vi "Move and Merge Element.vi"(7 "Direction":T2, 11 "Board Array":u8[][](array[numeric])) -> (1 "Game Status":T1, 2 "Score":i32, 3 "Board Array":u8[][](array[numeric]))   [LabVIEW 2020, in "Game.lvlib"]
uses:
  Game.lvlib
  Direction.ctl
  Game Status.ctl
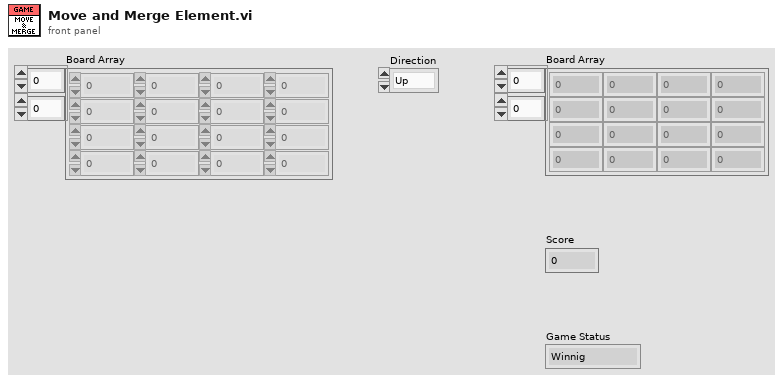
[diagram p1: front panel]
types:
  T1 = typedef "Game Status.ctl" = enum16{"Winnig", "Game Over", "Continute"}
  T2 = typedef "Direction.ctl" = enum16{"Up", "Down", "Left", "Right"}
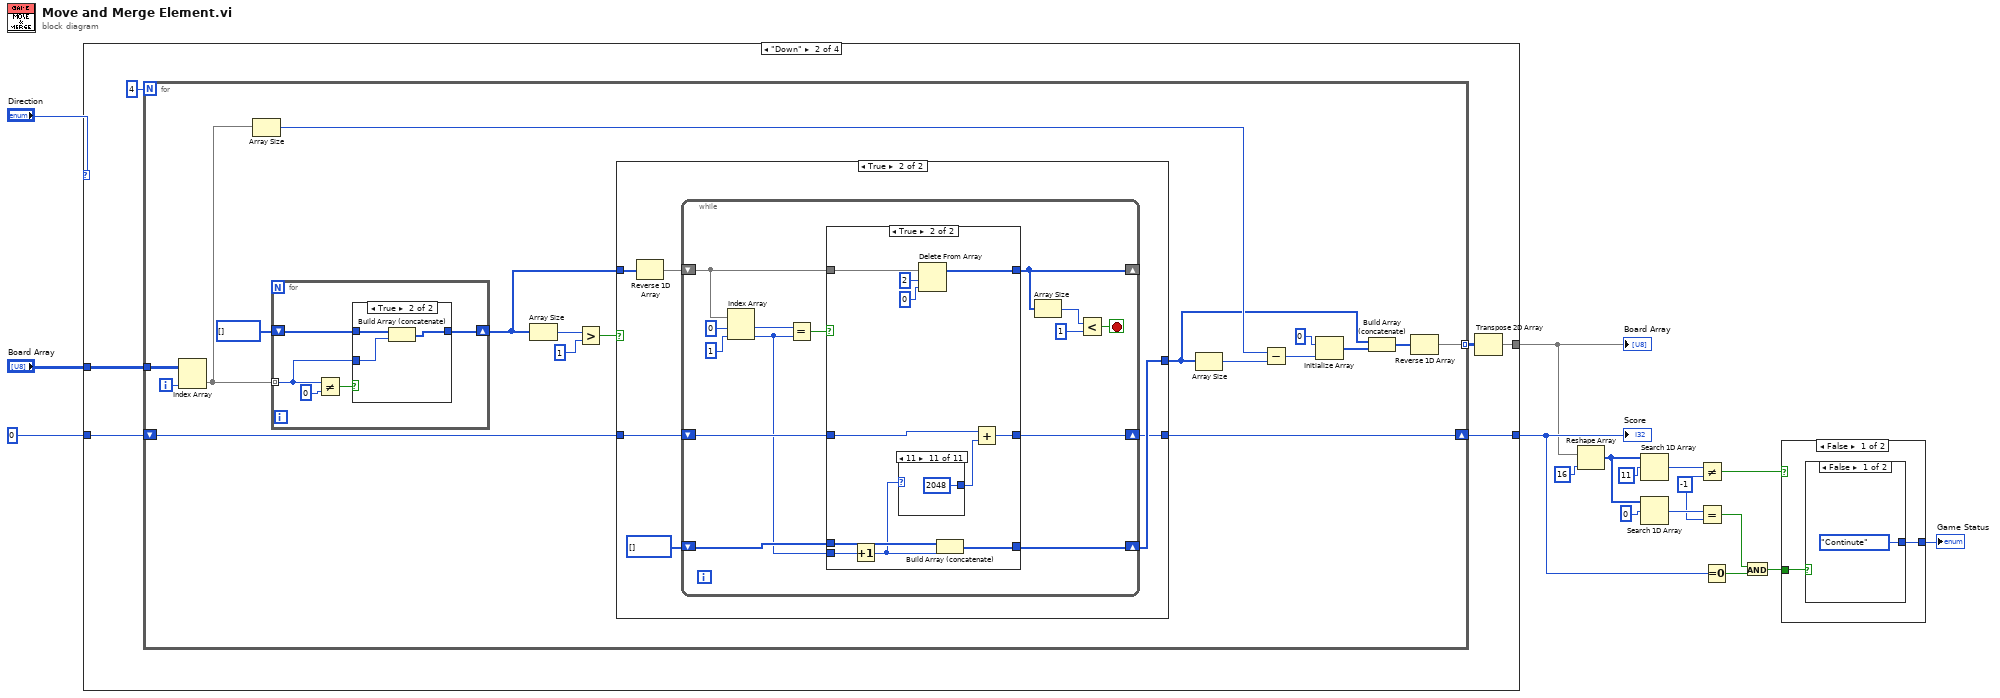
[diagram p0: block diagram]
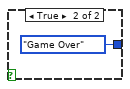
[diagram p2: hidden frame]
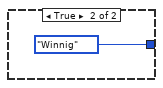
[diagram p3: hidden frame]
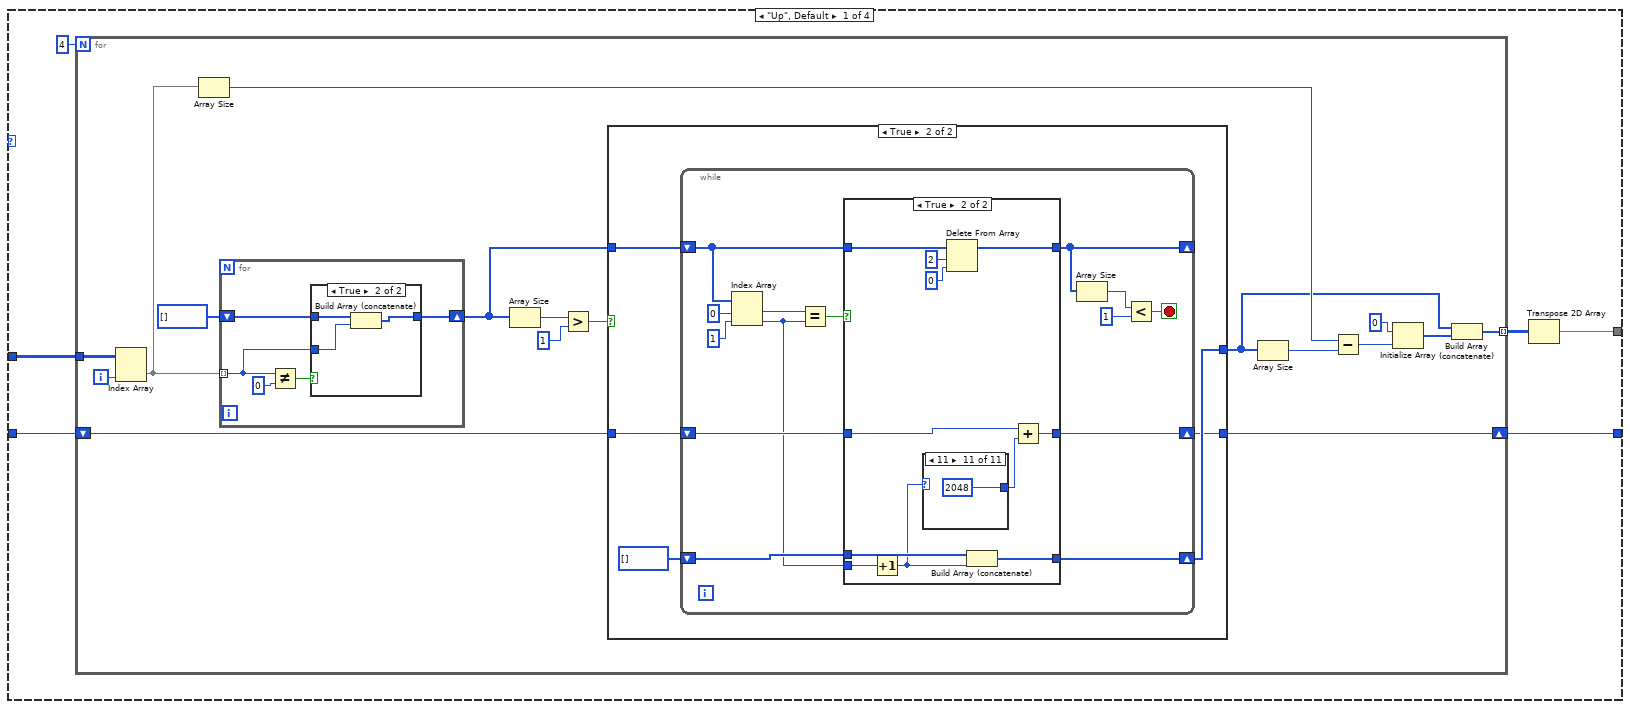
[diagram p4: hidden frame]
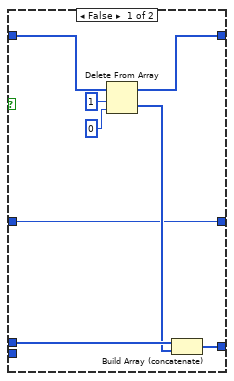
[diagram p6: hidden frame]
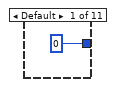
[diagram p7: hidden frame]
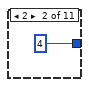
[diagram p8: hidden frame]
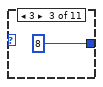
[diagram p9: hidden frame]
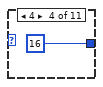
[diagram p10: hidden frame]
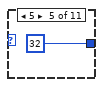
[diagram p11: hidden frame]
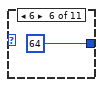
[diagram p12: hidden frame]
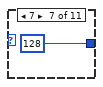
[diagram p13: hidden frame]
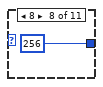
[diagram p14: hidden frame]
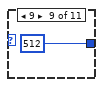
[diagram p15: hidden frame]
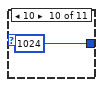
[diagram p16: hidden frame]
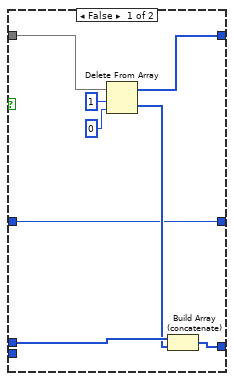
[diagram p19: hidden frame]
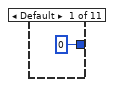
[diagram p20: hidden frame]
diagram:
  w1 = -1 ("y")
  n1 = case shown="\"Down\"" "Direction" {
    tunnel: "Board Array" -> [w23 w106 w190 w272]
    tunnel: [w18 w101 w188 w270] -> w2
    tunnel: [w20 w103 w187 w269] -> w13
    tunnel: 0 -> [w19 w102 w186 w268]
    frame "Up", Default {
      n2 = for {
        N: 4 -> [_]
        tunnel: w23 -> [w40]
        tunnel: [w25] -> w21 mode=indexing
        shift-right: [w28] -> w20
        shift-left: w19 -> [w27]
        i -> [w26]
        n3 = Index Array(array=w40, index (col)=w26) -> (element=w38:u8[])  [unwired: 1 in]
        n4 = Array Size(array=w38) -> (size(s)=w37:i32)
        n5 = for {
          tunnel: w38 -> [w94] mode=indexing
          shift-right: [w93] -> w32
          shift-left: u8[] [] -> [w92]
          n6 = Not Equal?(x=w94, y=u8 0) -> (x != y?=w95:bool)
          n7 = case shown="True" w95 {
            tunnel: w94 -> [_ w98]
            tunnel: [w97 w100] -> w93
            tunnel: w92 -> [w97 w99]
            frame False {
            }
            frame True {
              n8 = Build Array (concatenate)(w99, w98) -> (w100:u8[])
            }
          }
        }
        n9 = Array Size(array=w32) -> (size(s)=w31:i32)
        n10 = Greater?(x=w31, y=1) -> (0:w33:bool)
        n11 = case shown="True" w33 {
          tunnel: w32 -> [w42 w45]
          tunnel: [w42 w46] -> w30
          tunnel: [w41 w44] -> w28
          tunnel: w27 -> [w41 w43]
          frame False {
          }
          frame True {
            n12 = while {
              shift-right: [w48] -> _
              shift-left: w45 -> [w60]
              shift-right: [w56] -> w46
              shift-left: u8[] [] -> [w55]
              shift-right: [w51] -> w44
              shift-left: w43 -> [w50]
              stop <- w54 stop-if-true
              n13 = Index Array(array=w60, index #1=0 ("index"), index #2=1 ("index")) -> (element #1=w59:u8, element #2=w49:u8)
              n14 = Equal?(x=w59, y=w49) -> (x = y?=w61:bool)
              n15 = case shown="True" w61 {
                tunnel: w60 -> [w69 w79]
                tunnel: [w66 w76] -> w48
                tunnel: w49 -> [_ w80]
                tunnel: [w65 w75] -> w56
                tunnel: w55 -> [w64 w74]
                tunnel: [w62 w72] -> w51
                tunnel: w50 -> [w62 w73]
                frame False {
                  n16 = Delete From Array(array=w69, length=1, index=0) -> (deleted portion=w63:u8[], array with subset deleted=w66:u8[])
                  n17 = Build Array (concatenate)(w64, w63) -> (w65:u8[])
                }
                frame True {
                  n18 = Increment(x=w80) -> (x+1=w70:u8)
                  n19 = case shown="11" w70 {
                    tunnel: [0 4 8 16 32 64 128 256 512 1024 2048] -> w71
                    frame Default {
                    }
                    frame 2 {
                    }
                    frame 3 {
                    }
                    frame 4 {
                    }
                    frame 5 {
                    }
                    frame 6 {
                    }
                    frame 7 {
                    }
                    frame 8 {
                    }
                    frame 9 {
                    }
                    frame 10 {
                    }
                    frame 11 {
                    }
                  }
                  n20 = Delete From Array(array=w79, length=2, index=0) -> (array with subset deleted=w76:u8[])  [unwired: 1 out]
                  n21 = Build Array (concatenate)(w74, w70) -> (w75:u8[])
                  n22 = Add(x=w73, y=w71) -> (x+y=w72:i32)
                }
              }
              n23 = Array Size(array=w48) -> (size(s)=w52:i32)
              n24 = Less?(x=w52, y=1) -> (x < y?=w54:bool)
            }
          }
        }
        n25 = Array Size(array=w30) -> (size(s)=w24:i32)
        n26 = Subtract(x=w37, y=w24) -> (x-y=w29:i32)
        n27 = Initialize Array(u8 0, w29) -> (w35:u8[])
        n28 = Build Array (concatenate)(w30, w35) -> (w25:u8[])
      }
      n29 = Transpose 2D Array(2D array=w21) -> (transposed array=w18:u8[][])
    }
    frame "Down" {
      n30 = for {
        N: 4 -> [_]
        tunnel: w106 -> [w124]
        tunnel: [w111] -> w104 mode=indexing
        shift-right: [w110] -> w103
        shift-left: w102 -> [w109]
        i -> [w108]
        n31 = Index Array(array=w124, index (col)=w108) -> (element=w122:u8[])  [unwired: 1 in]
        n32 = Array Size(array=w122) -> (size(s)=w121:i32)
        n33 = for {
          tunnel: w122 -> [w179] mode=indexing
          shift-right: [w178] -> w116
          shift-left: u8[] [] -> [w177]
          n34 = Not Equal?(x=w179, y=u8 0) -> (x != y?=w180:bool)
          n35 = case shown="True" w180 {
            tunnel: w179 -> [_ w183]
            tunnel: [w182 w185] -> w178
            tunnel: w177 -> [w182 w184]
            frame False {
            }
            frame True {
              n36 = Build Array (concatenate)(w184, w183) -> (w185:u8[])
            }
          }
        }
        n37 = Array Size(array=w116) -> (size(s)=w115:i32)
        n38 = Greater?(x=w115, y=1) -> (0:w117:bool)
        n39 = case shown="True" w117 {
          tunnel: w116 -> [w126 w131]
          tunnel: [w126 w130] -> w114
          tunnel: [w125 w128] -> w110
          tunnel: w109 -> [w125 w127]
          frame False {
          }
          frame True {
            n40 = Reverse 1D Array(array=w131) -> (reversed array=w129:u8[])
            n41 = while {
              shift-right: [w133] -> _
              shift-left: w129 -> [w145]
              shift-right: [w141] -> w130
              shift-left: u8[] [] -> [w140]
              shift-right: [w136] -> w128
              shift-left: w127 -> [w135]
              stop <- w139 stop-if-true
              n42 = Index Array(array=w145, index #1=0 ("index"), index #2=1 ("index")) -> (element #1=w144:u8, element #2=w134:u8)
              n43 = Equal?(x=w144, y=w134) -> (x = y?=w146:bool)
              n44 = case shown="True" w146 {
                tunnel: w145 -> [w154 w164]
                tunnel: [w151 w161] -> w133
                tunnel: w134 -> [_ w165]
                tunnel: [w150 w160] -> w141
                tunnel: w140 -> [w149 w159]
                tunnel: [w147 w157] -> w136
                tunnel: w135 -> [w147 w158]
                frame False {
                  n45 = Delete From Array(array=w154, length=1, index=0) -> (deleted portion=w148:u8[], array with subset deleted=w151:u8[])
                  n46 = Build Array (concatenate)(w149, w148) -> (w150:u8[])
                }
                frame True {
                  n47 = Increment(x=w165) -> (x+1=w155:u8)
                  n48 = case shown="11" w155 {
                    tunnel: [0 4 8 16 32 64 128 256 512 1024 2048] -> w156
                    frame Default {
                    }
                    frame 2 {
                    }
                    frame 3 {
                    }
                    frame 4 {
                    }
                    frame 5 {
                    }
                    frame 6 {
                    }
                    frame 7 {
                    }
                    frame 8 {
                    }
                    frame 9 {
                    }
                    frame 10 {
                    }
                    frame 11 {
                    }
                  }
                  n49 = Delete From Array(array=w164, length=2, index=0) -> (array with subset deleted=w161:u8[])  [unwired: 1 out]
                  n50 = Build Array (concatenate)(w159, w155) -> (w160:u8[])
                  n51 = Add(x=w158, y=w156) -> (x+y=w157:i32)
                }
              }
              n52 = Array Size(array=w133) -> (size(s)=w137:i32)
              n53 = Less?(x=w137, y=1) -> (x < y?=w139:bool)
            }
          }
        }
        n54 = Array Size(array=w114) -> (size(s)=w107:i32)
        n55 = Subtract(x=w121, y=w107) -> (x-y=w113:i32)
        n56 = Initialize Array(u8 0, w113) -> (w119:u8[])
        n57 = Build Array (concatenate)(w114, w119) -> (w112:u8[])
        n58 = Reverse 1D Array(array=w112) -> (reversed array=w111:u8[])
      }
      n59 = Transpose 2D Array(2D array=w104) -> (transposed array=w101:u8[][])
    }
    frame "Left" {
      n60 = for {
        N: 4 -> [_]
        tunnel: w190 -> [w207]
        tunnel: [w194] -> w188 mode=indexing
        shift-right: [w193] -> w187
        shift-left: w186 -> [w192]
        i -> [w195]
        n61 = Index Array(array=w207, index (row)=w195) -> (element=w205:u8[])  [unwired: 1 in]
        n62 = Array Size(array=w205) -> (size(s)=w204:i32)
        n63 = for {
          tunnel: w205 -> [w261] mode=indexing
          shift-right: [w260] -> w199
          shift-left: u8[] [] -> [w259]
          n64 = Not Equal?(x=w261, y=u8 0) -> (x != y?=w262:bool)
          n65 = case shown="True" w262 {
            tunnel: w261 -> [_ w265]
            tunnel: [w264 w267] -> w260
            tunnel: w259 -> [w264 w266]
            frame False {
            }
            frame True {
              n66 = Build Array (concatenate)(w266, w265) -> (w267:u8[])
            }
          }
        }
        n67 = Array Size(array=w199) -> (size(s)=w198:i32)
        n68 = Greater?(x=w198, y=1) -> (0:w200:bool)
        n69 = case shown="True" w200 {
          tunnel: w199 -> [w209 w212]
          tunnel: [w209 w213] -> w197
          tunnel: [w208 w211] -> w193
          tunnel: w192 -> [w208 w210]
          frame False {
          }
          frame True {
            n70 = while {
              shift-right: [w215] -> _
              shift-left: w212 -> [w227]
              shift-right: [w223] -> w213
              shift-left: u8[] [] -> [w222]
              shift-right: [w218] -> w211
              shift-left: w210 -> [w217]
              stop <- w221 stop-if-true
              n71 = Index Array(array=w227, index #1=0 ("index"), index #2=1 ("index")) -> (element #1=w226:u8, element #2=w216:u8)
              n72 = Equal?(x=w226, y=w216) -> (x = y?=w228:bool)
              n73 = case shown="True" w228 {
                tunnel: w227 -> [w236 w246]
                tunnel: [w233 w243] -> w215
                tunnel: w216 -> [_ w247]
                tunnel: [w232 w242] -> w223
                tunnel: w222 -> [w231 w241]
                tunnel: [w229 w239] -> w218
                tunnel: w217 -> [w229 w240]
                frame False {
                  n74 = Delete From Array(array=w236, length=1, index=0) -> (deleted portion=w230:u8[], array with subset deleted=w233:u8[])
                  n75 = Build Array (concatenate)(w231, w230) -> (w232:u8[])
                }
                frame True {
                  n76 = Increment(x=w247) -> (x+1=w237:u8)
                  n77 = case shown="11" w237 {
                    tunnel: [0 4 8 16 32 64 128 256 512 1024 2048] -> w238
                    frame Default {
                    }
                    frame 2 {
                    }
                    frame 3 {
                    }
                    frame 4 {
                    }
                    frame 5 {
                    }
                    frame 6 {
                    }
                    frame 7 {
                    }
                    frame 8 {
                    }
                    frame 9 {
                    }
                    frame 10 {
                    }
                    frame 11 {
                    }
                  }
                  n78 = Delete From Array(array=w246, length=2, index=0) -> (array with subset deleted=w243:u8[])  [unwired: 1 out]
                  n79 = Build Array (concatenate)(w241, w237) -> (w242:u8[])
                  n80 = Add(x=w240, y=w238) -> (x+y=w239:i32)
                }
              }
              n81 = Array Size(array=w215) -> (size(s)=w219:i32)
              n82 = Less?(x=w219, y=1) -> (x < y?=w221:bool)
            }
          }
        }
        n83 = Array Size(array=w197) -> (size(s)=w191:i32)
        n84 = Subtract(x=w204, y=w191) -> (x-y=w196:i32)
        n85 = Initialize Array(u8 0, w196) -> (w202:u8[])
        n86 = Build Array (concatenate)(w197, w202) -> (w194:u8[])
      }
    }
    frame "Right" {
      n87 = for {
        N: 4 -> [_]
        tunnel: w272 -> [w290]
        tunnel: [w276] -> w270 mode=indexing
        shift-right: [w275] -> w269
        shift-left: w268 -> [w274]
        i -> [w277]
        n88 = Index Array(array=w290, index (row)=w277) -> (element=w288:u8[])  [unwired: 1 in]
        n89 = Array Size(array=w288) -> (size(s)=w287:i32)
        n90 = for {
          tunnel: w288 -> [w345] mode=indexing
          shift-right: [w344] -> w282
          shift-left: u8[] [] -> [w343]
          n91 = Not Equal?(x=w345, y=u8 0) -> (x != y?=w346:bool)
          n92 = case shown="True" w346 {
            tunnel: w345 -> [_ w349]
            tunnel: [w348 w351] -> w344
            tunnel: w343 -> [w348 w350]
            frame False {
            }
            frame True {
              n93 = Build Array (concatenate)(w350, w349) -> (w351:u8[])
            }
          }
        }
        n94 = Array Size(array=w282) -> (size(s)=w281:i32)
        n95 = Greater?(x=w281, y=1) -> (0:w283:bool)
        n96 = case shown="True" w283 {
          tunnel: w282 -> [w292 w297]
          tunnel: [w292 w296] -> w280
          tunnel: [w291 w294] -> w275
          tunnel: w274 -> [w291 w293]
          frame False {
          }
          frame True {
            n97 = Reverse 1D Array(array=w297) -> (reversed array=w295:u8[])
            n98 = while {
              shift-right: [w299] -> _
              shift-left: w295 -> [w311]
              shift-right: [w307] -> w296
              shift-left: u8[] [] -> [w306]
              shift-right: [w302] -> w294
              shift-left: w293 -> [w301]
              stop <- w305 stop-if-true
              n99 = Index Array(array=w311, index #1=0 ("index"), index #2=1 ("index")) -> (element #1=w310:u8, element #2=w300:u8)
              n100 = Equal?(x=w310, y=w300) -> (x = y?=w312:bool)
              n101 = case shown="True" w312 {
                tunnel: w311 -> [w320 w330]
                tunnel: [w317 w327] -> w299
                tunnel: w300 -> [_ w331]
                tunnel: [w316 w326] -> w307
                tunnel: w306 -> [w315 w325]
                tunnel: [w313 w323] -> w302
                tunnel: w301 -> [w313 w324]
                frame False {
                  n102 = Delete From Array(array=w320, length=1, index=0) -> (deleted portion=w314:u8[], array with subset deleted=w317:u8[])
                  n103 = Build Array (concatenate)(w315, w314) -> (w316:u8[])
                }
                frame True {
                  n104 = Increment(x=w331) -> (x+1=w321:u8)
                  n105 = case shown="11" w321 {
                    tunnel: [0 4 8 16 32 64 128 256 512 1024 2048] -> w322
                    frame Default {
                    }
                    frame 2 {
                    }
                    frame 3 {
                    }
                    frame 4 {
                    }
                    frame 5 {
                    }
                    frame 6 {
                    }
                    frame 7 {
                    }
                    frame 8 {
                    }
                    frame 9 {
                    }
                    frame 10 {
                    }
                    frame 11 {
                    }
                  }
                  n106 = Delete From Array(array=w330, length=2, index=0) -> (array with subset deleted=w327:u8[])  [unwired: 1 out]
                  n107 = Build Array (concatenate)(w325, w321) -> (w326:u8[])
                  n108 = Add(x=w324, y=w322) -> (x+y=w323:i32)
                }
              }
              n109 = Array Size(array=w299) -> (size(s)=w303:i32)
              n110 = Less?(x=w303, y=1) -> (x < y?=w305:bool)
            }
          }
        }
        n111 = Array Size(array=w280) -> (size(s)=w273:i32)
        n112 = Subtract(x=w287, y=w273) -> (x-y=w279:i32)
        n113 = Initialize Array(u8 0, w279) -> (w285:u8[])
        n114 = Build Array (concatenate)(w280, w285) -> (w278:u8[])
        n115 = Reverse 1D Array(array=w278) -> (reversed array=w276:u8[])
      }
    }
  }
  "Board Array" <- w2
  "Score" <- w13
  n116 = Reshape Array(w2, 16 ("dimension size")) -> (w6:u8[])
  n117 = Search 1D Array(1D array=w6, element=u8 11) -> (index of element=w8:i32)  [unwired: 1 in]
  n118 = Search 1D Array(1D array=w6, element=u8 0) -> (index of element=w4:i32)  [unwired: 1 in]
  n119 = Not Equal?(x=w8, y=w1) -> (x != y?=w7:bool)
  n120 = Equal?(x=w4, y=w1) -> (x = y?=w3:bool)
  n121 = Equal To 0?(x=w13) -> (x = 0?=w12:bool)
  n122 = And(x=w3, y=w12) -> (x .and. y?=w10:bool)
  n123 = case shown="False" w7 {
    tunnel: [w352 Game_Status."Winnig" ("Game Status")] -> w14
    tunnel: w10 -> [w353 _]
    frame False {
      n124 = case shown="False" w353 {
        tunnel: [Game_Status."Continute" ("Game Status") Game_Status."Game Over" ("Game Status")] -> w352
        frame False {
        }
        frame True {
        }
      }
    }
    frame True {
    }
  }
  "Game Status" <- w14
